vi "GT 2D Compare Data.vi"(6 "fifo":i16, 7 "pBuf":cluster{"px":i32, "py":i32}[](array[cluster]), 8 "error in (no error)":errorcluster caption="错误输入（无错误）", 9 "count":i16, 10 "chn":i16, 11 "cardNum":i16) -> (0 "error out":errorcluster caption="错误输出", 3 "function return":i16, 5 "pBuf out":cluster{"px":i32, "py":i32}[](array[cluster]))   [LabVIEW 2014, in "gts.lvlib"]
doc: "GT_API GT_2DCompareData(short cardNum,short chn,short count,T2DCompareData *pBuf,short fifo);"
uses:
  gts.lvlib
  gts.dll
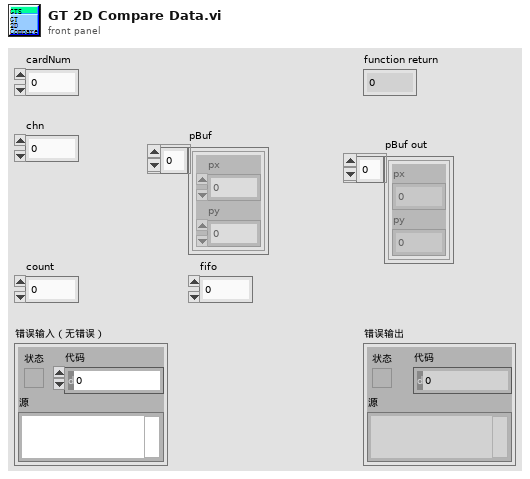
[diagram p1: front panel]
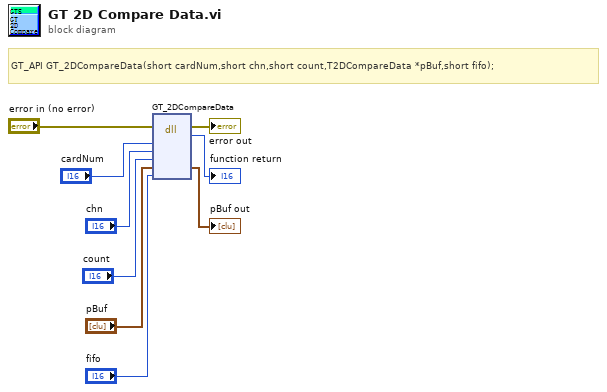
[diagram p0: block diagram]
diagram:
  # "GT_API GT_2DCompareData(short cardNum,short chn,short count,T2DCompareData *pBuf,short fifo);"
  n1 = dll-call lib="PTH2?abs D\t王淼清$控制卡常用功能例程(Labview)gts.*" fn="GT_2DCompareData"(error in="error in (no error)", "cardNum"="cardNum", "chn"="chn", "count"="count", "pBuf"="pBuf", "fifo"="fifo") -> (error out=→"error out":errorcluster, "返回类型"=→"function return":i16, "pBuf"=→"pBuf out":cluster{"px":i32, "py":i32}[])  [unwired: 6 in, 1 out]
